vi "Mass Rename Window Titles.vi"() -> ()   [LabVIEW 2023]
panel:
  out "VIs Total":i32
  out "VIs Processed":i32
  in  "Replace String":string
  in  "Search String":string
  in  "Folder":path
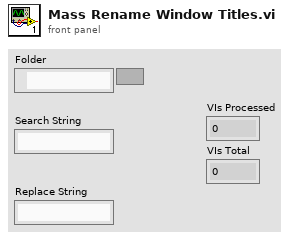
[diagram p1: front panel]
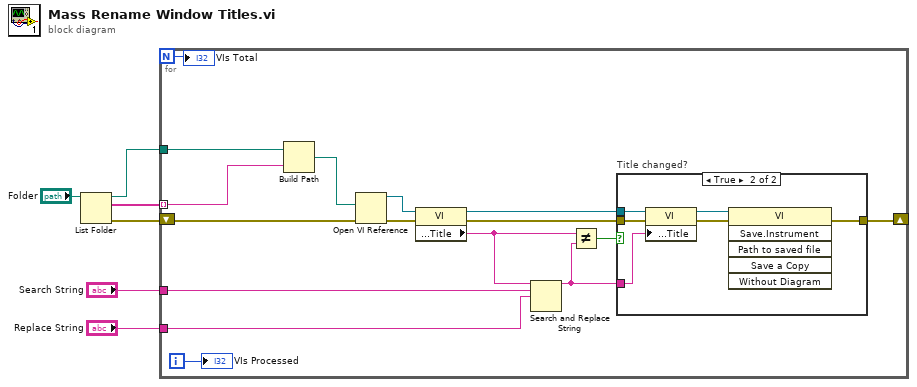
[diagram p0: block diagram]
diagram:
  n1 = List Folder(path="Folder") -> (path out=w4:path, filenames=w5:string[], error out=w3:errorcluster)  [unwired: 3 in, 1 out]
  n2 = for {
    N -> [w7]
    tunnel: w5 -> [w21] mode=indexing
    tunnel: w4 -> [w22]
    tunnel: "Search String" -> [w16]
    tunnel: "Replace String" -> [w15]
    shift-right: [w12] -> _
    shift-left: w3 -> [w20]
    i -> [w8]
    n3 = Build Path(base path=w22, name or relative path=w21) -> (appended path=w19:path)
    n4 = Open VI Reference(vi path=w19, error in (no error)=w20) -> (vi reference=w18:refnum<vi>, error out=w14:errorcluster)  [unwired: 4 in]
    n5 = property class="VI"(reference=w18, error in=w14) -> (reference out=w17:refnum<vi>, error out=w13:errorcluster, "Front Panel.Title"=w10:string)
    n6 = Search and Replace String(input string=w10, search string=w16, replace string=w15) -> (result string=w11:string)  [unwired: 5 in, 3 out]
    n7 = Not Equal?(x=w10, y=w11) -> (x != y?=w9:bool)
    n8 = case "Title changed?" shown="True" w9 {
      tunnel: w17 -> [_ w29]
      tunnel: w13 -> [w23 w27]
      tunnel: [w23 w25] -> w12
      tunnel: w11 -> [_ w24]
      frame False {
      }
      frame True {
        n9 = property class="VI"(reference=w29, error in=w27, "Front Panel.Title"=w24) -> (reference out=w28:refnum<vi>, error out=w26:errorcluster)
        n10 = invoke class="VI" method="Save.Instrument"(reference=w28, error in=w26) -> (error out=w25:errorcluster)  [unwired: 4 in, 5 out]
      }
    }
    "VIs Processed" <- w8
    "VIs Total" <- w7
  }
